vi "FTW-Listener-Construct.vi"(0 "Gmsg_Listener In":refnum<class "FTW-Listener.lvclass">, 5 "Address":string, 11 "error in":errorcluster) -> (4 "Gmsg_Listener Out":refnum<class "FTW-Listener.lvclass">, 15 "error out":errorcluster)   [LabVIEW 2013, in "FTW-Listener.lvclass"]
uses:
  FTW-Listener.lvclass
  FTW-Listener.lvclass/FTW-Listener.ctl
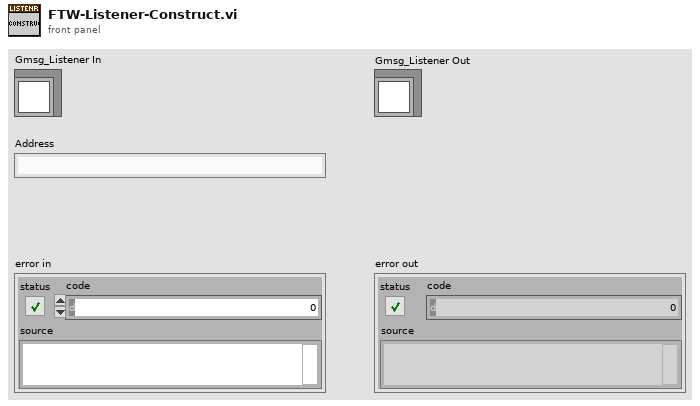
[diagram p1: front panel]
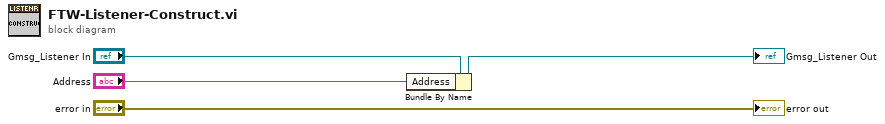
[diagram p0: block diagram]
diagram:
  n1 = Bundle By Name(cluster="Gmsg_Listener In", "Address"="Address") -> (→"Gmsg_Listener Out":refnum<class "FTW-Listener.lvclass">)
  "error out" <- "error in"
